vi "tcp shot sender send data.vi"(8 "error in (no error)":errorcluster, 11 "Data in":T3) -> (0 "error out":errorcluster, 3 "Data out":T3)   [LabVIEW 2020]
uses:
  tcp shot sender queue.ctl
  TCP Multiple Connections State.ctl
panel:
  out "error out 2":errorcluster
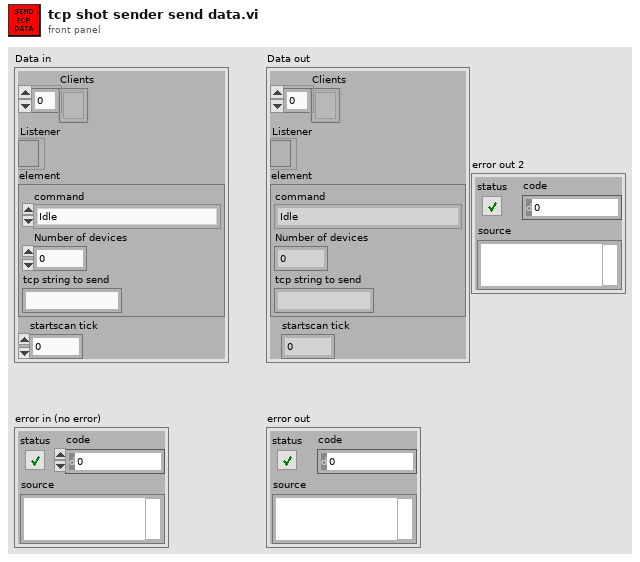
[diagram p1: front panel]
types:
  T1 = typedef "tcp shot sender queue.ctl" = cluster{"command":T2, "Number of devices":i32, "tcp string to send":string}
  T2 = typedef "TCP Multiple Connections State.ctl" = enum16{"Idle", "Initialize", "Start Scan", "Send Data", "Stop", "End Scan"}
  T3 = cluster{"Clients":refnum<k5>[], "Listener":refnum<k5>, "element":T1, "startscan tick":u32}
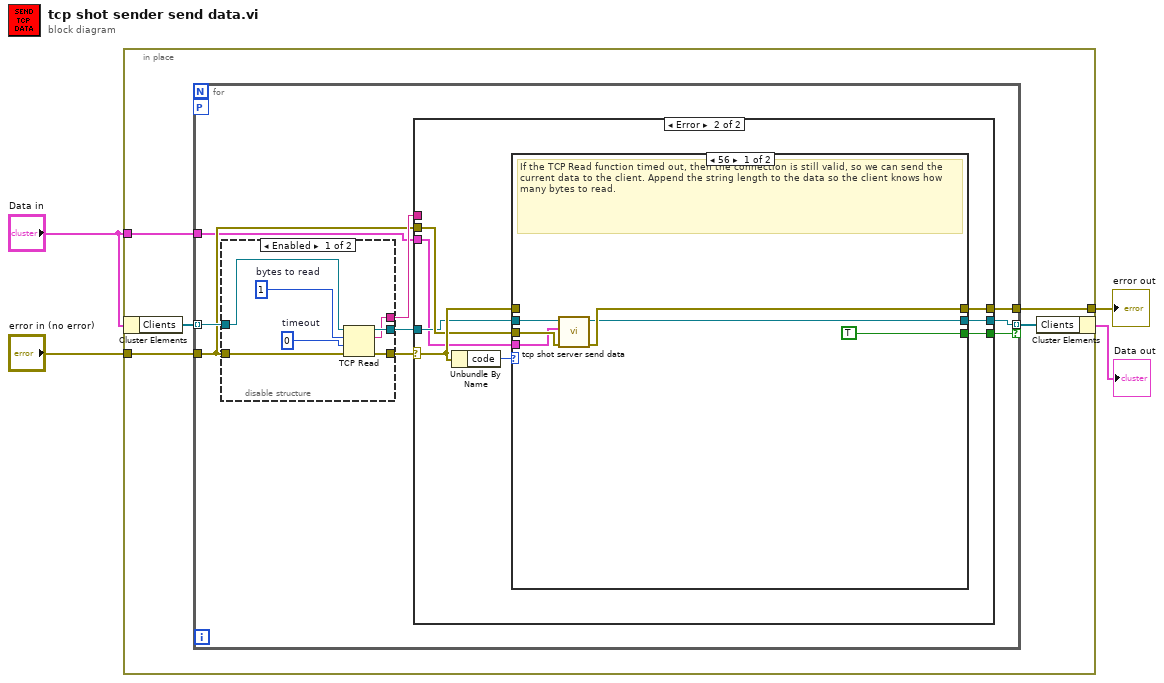
[diagram p0: block diagram]
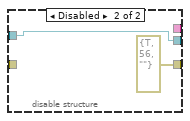
[diagram p2: hidden frame]
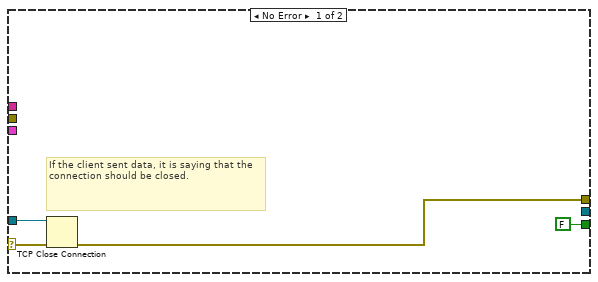
[diagram p3: hidden frame]
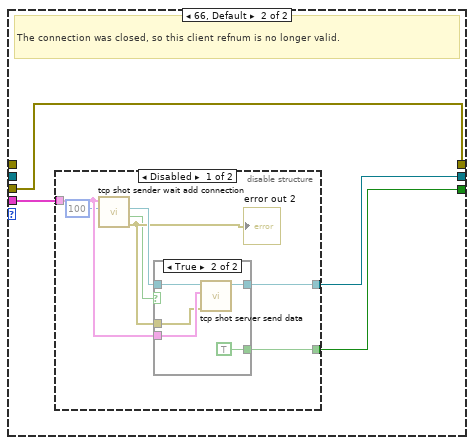
[diagram p4: hidden frame]
diagram:
  n1 = in-place {
    in-place-border: "error in (no error)" -> [w9]
    in-place-border: [w8] -> w4
    in-place-border: "Data in" -> [w5]
    n2 = in-place-cluster #1("Data in") -> ("Clients"=w7:refnum<k5>[])
    n3 = for {
      tunnel: w7 -> [w18] mode=indexing
      tunnel: [w14] -> w6 mode=indexing if=w13
      tunnel: w5 -> [w10]
      tunnel: w9 -> [w11]
      tunnel: [w12] -> w8
      workers-P: _ -> [_]
      n4 = disable-structure shown="Enabled" {
        disable-tunnel: w18 -> [w25 w27]
        disable-tunnel: [w24 w27] -> w17
        disable-tunnel: [w21 errorcluster {"status"=TRUE, "code"=56, "source"=""} ("error out")] -> w16
        disable-tunnel: [w20 _] -> w15
        disable-tunnel: w11 -> [w19 _]
        frame Enabled {
          w22 = 0  # timeout
          w23 = 1  # bytes to read
          n5 = TCP Read(connection ID=w25, bytes to read=w23, error in (no error)=w19, 9:w22) -> (connection ID out=w24:refnum<k5>, data out=w20:string, error out=w21:errorcluster)  [unwired: 1 out]
        }
        frame Disabled {
        }
      }
      n6 = case shown="Error" w16 {
        selector: w16 -> [w30 w38]
        tunnel: w17 -> [w31 w35]
        tunnel: w15 -> [_ _]
        tunnel: [_ w33] -> w14
        tunnel: [FALSE w34] -> w13
        tunnel: [w28 w37] -> w12
        tunnel: w11 -> [_ w36]
        tunnel: w10 -> [_ w32]
        frame No Error {
          # "If the client sent data, it is saying that the connection should be closed."
          # "If the client sent data, it is saying that the connection should be closed."
          n7 = TCP Close Connection(connection ID=w31, error in (no error)=w30) -> (error out=w28:errorcluster)  [unwired: 2 out]
        }
        frame Error {
          # "Ignore connection closed and timeout errors"
          n8 = Unbundle By Name(w38) -> ("code"=w39:i32)
          n9 = case shown="56" w39 {
            tunnel: w38 -> [_ _]
            tunnel: [w45 w49] -> w37
            tunnel: w36 -> [w41 w49]
            tunnel: w35 -> [w44 _]
            tunnel: [TRUE w48] -> w34
            tunnel: [w43 w46] -> w33
            tunnel: w32 -> [w40 w47]
            frame 56 {
              # "If the TCP Read function timed out, then the connection is still valid, so we can send the current data to the client. Append the string length to the data so the client knows how many bytes to read."
              n10 = call "tcp shot server send data.vi"("error in (no error)"=w41, "Data in"=w40, "TCP Network Connection in"=w44) -> ("error out"=w45:errorcluster, "TCP Network Connection out"=w43:refnum<k5>)  [unwired: 7 in]
            }
            frame 66, Default {
              # "The connection was closed, so this client refnum is no longer valid."
              n11 = disable-structure shown="Disabled" {
                disable-tunnel: [w51 _] -> w48
                disable-tunnel: w47 -> [w54 _]
                disable-tunnel: [w55 _] -> w46
                frame Disabled {
                  n12 = call "tcp shot sender wait add connection.vi"("timeout ms"=100, "Data in"=w54) -> ("error out"=w53:errorcluster, "connected"=w52:bool, "connection ID"=w56:refnum<k5>)  [unwired: 6 in, 1 out]
                  "error out 2" <- w53
                  n13 = case shown="True" w52 {
                    tunnel: w56 -> [w57 w62]
                    tunnel: [w57 w61] -> w55
                    tunnel: w54 -> [_ w60]
                    tunnel: w53 -> [_ w59]
                    tunnel: [_ TRUE] -> w51
                    frame False {
                    }
                    frame True {
                      n14 = call "tcp shot server send data.vi"("error in (no error)"=w59, "Data in"=w60, "TCP Network Connection in"=w62) -> ("TCP Network Connection out"=w61:refnum<k5>)  [unwired: 7 in, 1 out]
                    }
                  }
                }
                frame Enabled {
                  # "reconnecting makes no sense\nif shot was missed too late\nscan has to end"
                }
              }
            }
          }
        }
      }
    }
    n15 = in-place-cluster #1("Clients"=w6) -> (→"Data out":T3)
  }
  "error out" <- w4
